vi "assOrAddLandmark.vi"(6 "noFoundLandmarks":i32, 8 "foundLandmarks":T1, 9 "noMeasurements":i32, 10 "measurements":dbl[][](array[numeric]), 11 "X":dbl[](array[numeric])) -> (0 "associatedLandmarks":i32[](array[numeric]), 1 "newLandmarks":dbl[][](array[numeric]), 2 "reObservedLandmarksRaB":dbl[][](array[numeric]), 3 "currentLandmarks":dbl[][](array[numeric]), 4 "noNewLandmarks":i32, 5 "noReObservedLandmarks":i32)   [LabVIEW 2009, in "LV_SLAM.lvlib"]
uses:
  LV_SLAM.lvlib
  <vilib>/Analysis/Matrix/Datatypes/RealMatrix.ctl
  <vilib>/Analysis/Matrix/Numeric/Conversions/Array To Matrix - RA2.vi
  <vilib>/Analysis/Matrix/NI_Matrix.lvlib
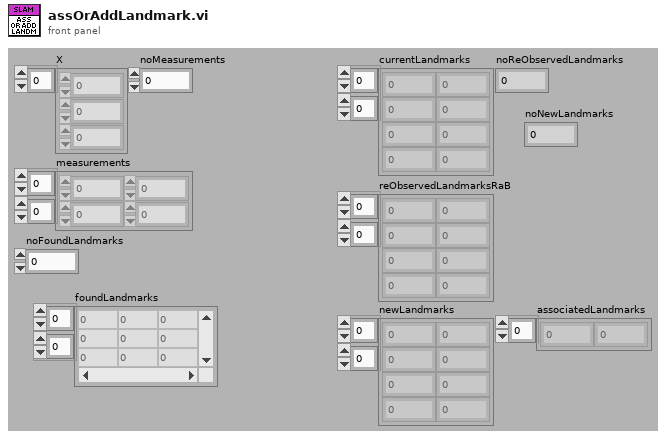
[diagram p1: front panel]
types:
  T1 = typedef "NI_Matrix.lvlib/RealMatrix.ctl" = dbl[][]
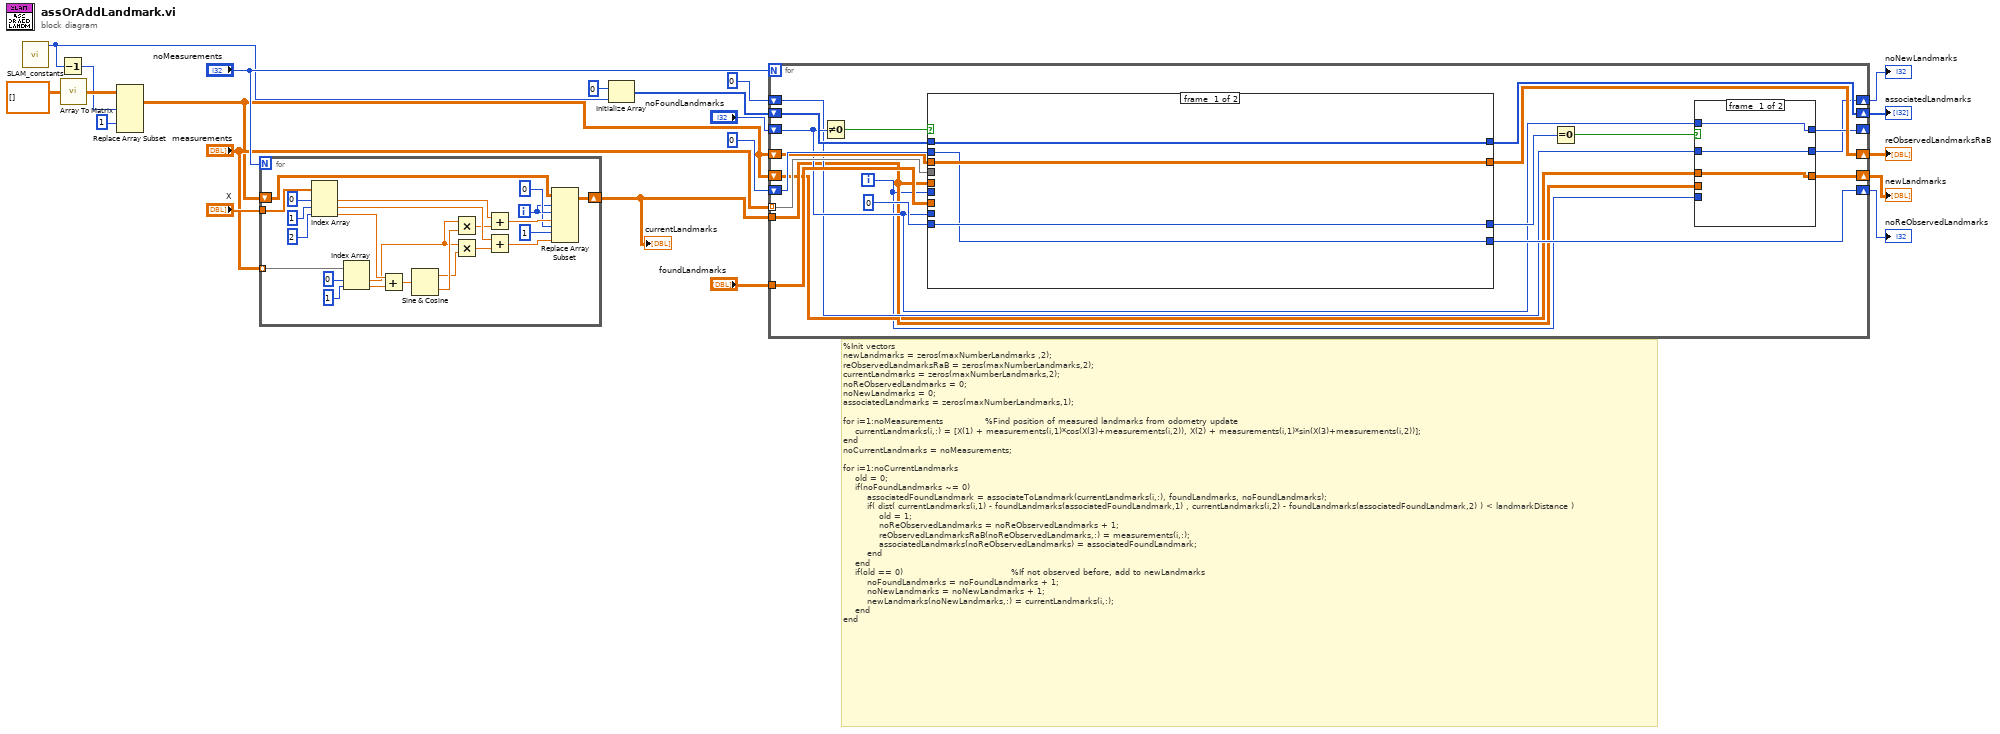
[diagram p0: block diagram]
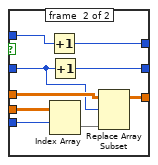
[diagram p2: hidden frame]
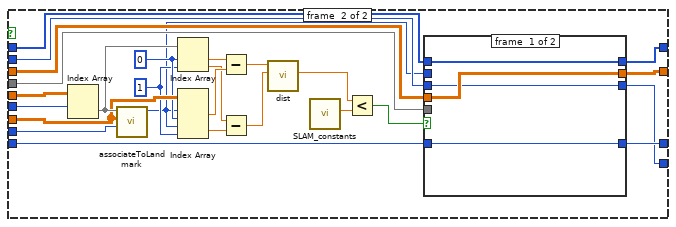
[diagram p3: hidden frame]
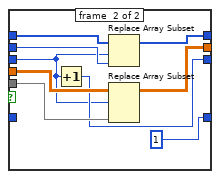
[diagram p4: hidden frame]
diagram:
  # "%Init vectors\nnewLandmarks = zeros(maxNumberLandmarks ,2);\nreObservedLandmarksRaB = zeros(maxNumberLandmarks,2);\ncurrentLandmarks = zeros(maxNumberLandmarks,2);\nnoReObservedLandmarks = 0;\nnoNewLandmarks = 0;\nassociatedLandmarks = zeros(maxNumberLandmarks,1);\n\nfor i=1:noMeasurements              %Find position of measured landmarks from odometry update\n    currentLandmarks(i,:) = [X(1) + measurements(i,1)*cos(X(3)+measurements(i,2)), X(2) + measurements(i,1)*sin(X(3)+measurements(i,2))];\nend\nnoCurrentLandmarks = noMeasurements;\n\nfor i=1:noCurrentLandmarks\n    old = 0;\n    if(noFoundLandmarks ~= 0)\n        associatedFoundLandmark = associateToLandmark(currentLandmarks(i,:), foundLandmarks, noFoundLandmarks);\n        if( dist( currentLandmarks(i,1) - foundLandmarks(associatedFoundLandmark,1) , currentLandmarks(i,2) - foundLandmarks(associatedFoundLandmark,2) ) < landmarkDistance )\n            old = 1;\n            noReObservedLandmarks = noReObservedLandmarks + 1;\n            reObservedLandmarksRaB(noReObservedLandmarks,:) = measurements(i,:);\n            associatedLandmarks(noReObservedLandmarks) = associatedFoundLandmark;\n        end\n    end\n    if(old == 0)                                    %If not observed before, add to newLandmarks\n        noFoundLandmarks = noFoundLandmarks + 1;\n        noNewLandmarks = noNewLandmarks + 1;\n        newLandmarks(noNewLandmarks,:) = currentLandmarks(i,:);\n    end\nend"
  n1 = call "SLAM_constants.vi"() -> ("maxNumberLandmarks"=w10:i32)  [unwired: 7 in, 4 out]
  n2 = Decrement(x=w10) -> (x-1=w18:i32)
  n3 = call-poly <vilib>:"Array To Matrix.vi"("Real 2D Array"=dbl[][] [] ("foundLandmarks")) -> ("Real Matrix"=w21:T1)
  n4 = Replace Array Subset(array=w21, index (dim 1)=w18, index (dim 3)=1 ("column N")) -> (w7:T1)  [unwired: 3 in]
  n5 = for {
    N: "noMeasurements" -> [_]
    tunnel: "X" -> [w45]
    tunnel: "measurements" -> [w40] mode=indexing
    shift-right: [w32] -> w1
    shift-left: w7 -> [w33]
    i -> [w27]
    n6 = Index Array(array=w45, index #1=0 ("index"), index #2=1 ("index"), index #3=2 ("index")) -> (element #1=w35:dbl, element #2=w34:dbl, element #3=w41:dbl)
    n7 = Index Array(array=w40, index #1=0 ("index"), index #2=1 ("index")) -> (element #1=w24:dbl, element #2=w37:dbl)
    n8 = Add(x=w41, y=w37) -> (x+y=w36:dbl)
    n9 = Sine & Cosine(0:w36) -> (1:w22:dbl, 2:w26:dbl)
    n10 = Multiply(x=w24, y=w26) -> (x*y=w25:dbl)
    n11 = Multiply(x=w24, y=w22) -> (x*y=w23:dbl)
    n12 = Add(x=w35, y=w25) -> (x+y=w29:dbl)
    n13 = Add(x=w34, y=w23) -> (x+y=w28:dbl)
    n14 = Replace Array Subset(array=w33, new element #1=w29, index (row) #1=w27, index (col) #1=0 ("index"), new element #2=w28, index (row) #2=w27, index (col) #2=1 ("index")) -> (w32:T1)
  }
  "currentLandmarks" <- w1
  n15 = Initialize Array(0 ("element"), w10) -> (w9:i32[])
  n16 = for {
    N: "noMeasurements" -> [_]
    tunnel: w1 -> [w49]
    tunnel: "foundLandmarks" -> [w64]
    shift-right: [w61] -> w2
    shift-left: 0 ("noReObservedLandmarks") -> [w62]
    tunnel: "measurements" -> [w59] mode=indexing
    shift-right: [w58] -> w3
    shift-left: w7 -> [w60]
    shift-right: [w56] -> w4
    shift-left: w9 -> [w57]
    shift-right: [w52] -> _
    shift-left: "noFoundLandmarks" -> [w53]
    shift-right: [w50] -> w5
    shift-left: 0 ("noNewLandmarks") -> [w51]
    shift-right: [w47] -> w6
    shift-left: w7 -> [w48]
    i -> [w46]
    n17 = Not Equal To 0?(x=w53) -> (x != 0?=w65:bool)
    n18 = case shown="True" w65 {
      tunnel: w49 -> [_ w107]
      tunnel: w64 -> [_ w103]
      tunnel: w46 -> [_ w106]
      tunnel: w53 -> [_ w105]
      tunnel: 0 ("index") -> [w81 w91]
      tunnel: [w81 w90] -> w54
      tunnel: w62 -> [w79 w89]
      tunnel: [w79 w88] -> w61
      tunnel: w60 -> [w80 w87]
      tunnel: w59 -> [_ w86]
      tunnel: [w80 w85] -> w58
      tunnel: w57 -> [w78 w84]
      tunnel: [w78 w82] -> w56
      frame #0 {
      }
      frame #1 {
        w101 = 1 ("index")
        w102 = 0 ("index")
        n19 = Index Array(array=w107, index (row)=w106) -> (element=w104:dbl[])  [unwired: 1 in]
        n20 = call "associateToLandmark.vi"("noFoundLandmarks"=w105, "foundLandmarks"=w103, "currentLandmark"=w104) -> ("associatedFoundLandmark"=w83:i32)  [unwired: 8 in]
        n21 = Index Array(array=w104, index #1=w102, index #2=w101) -> (element #1=w100:dbl, element #2=w98:dbl)
        n22 = Index Array(array=w103, index (row) #1=w83, index (col) #1=w102, index (row) #2=w83, index (col) #2=w101) -> (element #1=w99:dbl, element #2=w97:dbl)
        n23 = Subtract(x=w100, y=w99) -> (x-y=w96:dbl)
        n24 = Subtract(x=w98, y=w97) -> (x-y=w95:dbl)
        n25 = call "dist.vi"("y"=w95, "x"=w96) -> ("d"=w94:dbl)  [unwired: 9 in]
        n26 = call "SLAM_constants.vi"() -> ("landmarkDistance"=w93:dbl)  [unwired: 7 in, 4 out]
        n27 = Less?(x=w94, y=w93) -> (x < y?=w92:bool)
        n28 = case shown="True" w92 {
          tunnel: w91 -> [w111 _]
          tunnel: [w111 1 ("index")] -> w90
          tunnel: w89 -> [w109 w112]
          tunnel: [w109 w114] -> w88
          tunnel: w87 -> [w110 w119]
          tunnel: w86 -> [_ w118]
          tunnel: [w110 w117] -> w85
          tunnel: w84 -> [w108 w116]
          tunnel: w83 -> [_ w115]
          tunnel: [w108 w113] -> w82
          frame #0 {
          }
          frame #1 {
            n29 = Increment(x=w112) -> (x+1=w114:i32)
            n30 = Replace Array Subset(array=w116, new element=w115, index=w112) -> (w113:i32[])
            n31 = Replace Array Subset(array=w119, new element=w118, index (row)=w112) -> (w117:T1)  [unwired: 1 in]
          }
        }
      }
    }
    n32 = Equal To 0?(x=w54) -> (x = 0?=w55:bool)
    n33 = case shown="True" w55 {
      tunnel: w53 -> [w68 w77]
      tunnel: [w68 w76] -> w52
      tunnel: w51 -> [w67 w69]
      tunnel: [w67 w74] -> w50
      tunnel: w49 -> [_ w73]
      tunnel: w48 -> [w66 w75]
      tunnel: [w66 w70] -> w47
      tunnel: w46 -> [_ w72]
      frame #0 {
      }
      frame #1 {
        n34 = Increment(x=w77) -> (x+1=w76:i32)
        n35 = Increment(x=w69) -> (x+1=w74:i32)
        n36 = Index Array(array=w73, index (row)=w72) -> (element=w71:dbl[])  [unwired: 1 in]
        n37 = Replace Array Subset(array=w75, new element=w71, index (row)=w69) -> (w70:T1)  [unwired: 1 in]
      }
    }
  }
  "reObservedLandmarksRaB" <- w3
  "newLandmarks" <- w6
  "noNewLandmarks" <- w5
  "noReObservedLandmarks" <- w2
  "associatedLandmarks" <- w4
